vi "MU Set Param.vi"(7 "writeVerify":u32, 8 "error in (no error)":errorcluster, 9 "value":u64, 10 "parameter":u32, 11 "handle":u64) -> (0 "error out (no error)":errorcluster, 3 "function return":u32)   [LabVIEW 2017, in "MU_3SL_interface.lvlib"]
uses:
  MU_3SL_interface.lvlib
  lib/MU_3SL_interface.dll
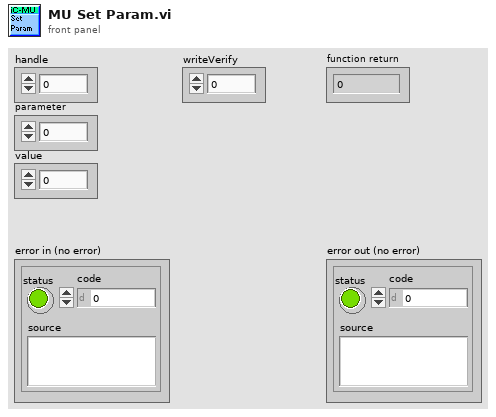
[diagram p1: front panel]
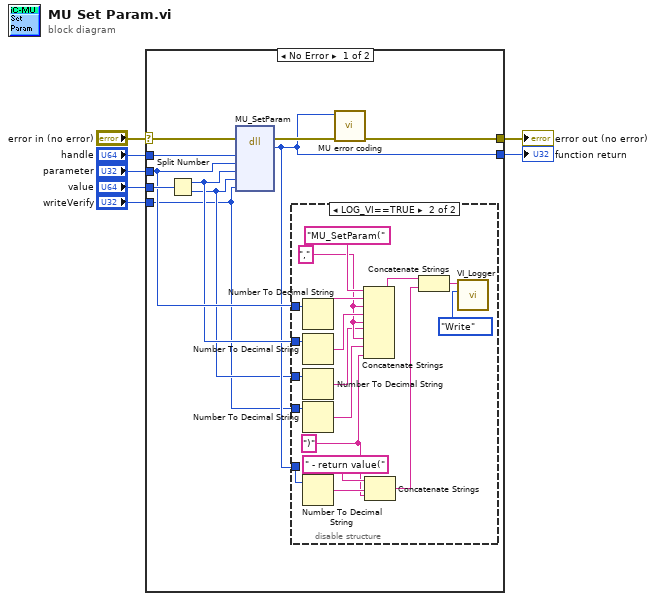
[diagram p0: block diagram]
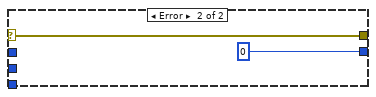
[diagram p3: hidden frame]
diagram:
  n1 = case shown="No Error" "error in (no error)" {
    selector: "error in (no error)" -> [w13 w37]
    tunnel: [w10 u32 0] -> w7
    tunnel: "handle" -> [w17 _]
    tunnel: "parameter" -> [w12 _]
    tunnel: "writeVerify" -> [w8 _]
    tunnel: [w15 w37] -> w3
    tunnel: "value" -> [w14 _]
    frame No Error {
      n2 = Split Number(x=w14) -> (hi(x)=w11:u32, lo(x)=w9:u32)
      n3 = dll-call lib="C:/Users/bes/AppData/Roaming/work/mu_9so/icsubmodules/soft_mu_3sl_master/lv_interface/lib/MU_3SL_interface**.*" fn="MU_SetParam"(error in=w13, "handle"=w17, "parameter"=w12, "valueHigh"=w11, "valueLow"=w9, "writeVerify"=w8) -> (error out=w16:errorcluster, "return type"=w10:u32)  [unwired: 7 in, 1 out]
      n4 = disable-structure shown="LOG_VI==TRUE" {
        disable-tunnel: w10 -> [_ w33]
        disable-tunnel: w12 -> [_ w28]
        disable-tunnel: w11 -> [_ w26]
        disable-tunnel: w9 -> [_ w23]
        disable-tunnel: w8 -> [_ w20]
        frame condition #0 {
        }
        frame condition #1 (active) {
          w18 = ")" ("string")
          w22 = "," ("string")
          n5 = Number To Decimal String(number=w28) -> (decimal integer string=w27:string)  [unwired: 1 in]
          n6 = Number To Decimal String(number=w26) -> (decimal integer string=w25:string)  [unwired: 1 in]
          n7 = Number To Decimal String(number=w23) -> (decimal integer string=w21:string)  [unwired: 1 in]
          n8 = Number To Decimal String(number=w20) -> (decimal integer string=w19:string)  [unwired: 1 in]
          n9 = Number To Decimal String(number=w33) -> (decimal integer string=w32:string)  [unwired: 1 in]
          n10 = Concatenate Strings("MU_SetParam(" ("Info in"), w27, w22, w25, w22, w21, w22, w19, w18) -> (w31:string)
          n11 = Concatenate Strings(" - return value(" ("string"), w32, w18) -> (w30:string)
          n12 = Concatenate Strings(w31, w30) -> (w29:string)
          n13 = call "VI_Logger.vi"("Action (Read)"=enum16{"Write", "Read"}."Write", "Info in"=w29) -> ()  [unwired: 8 in, 2 out]
        }
      }
      n14 = call "MU error coding.vi"("error in (no error)"=w16, "function return in"=w10) -> ("error out"=w15:errorcluster)  [unwired: 9 in]
    }
    frame Error {
    }
  }
  "function return" <- w7
  "error out (no error)" <- w3
